vi "lib1.vi"() -> ()   [LabVIEW 2013]
panel:
  out "year of study":i32
  out "Month":i32
  out "number":i32
  out "year":i32
  out "date string":string
  out "id number":i32
  out "offset string rollnumber":string
  out "Roll Number string":string
  out "Image Out":T1(plugin-control)
  in  "stop":bool
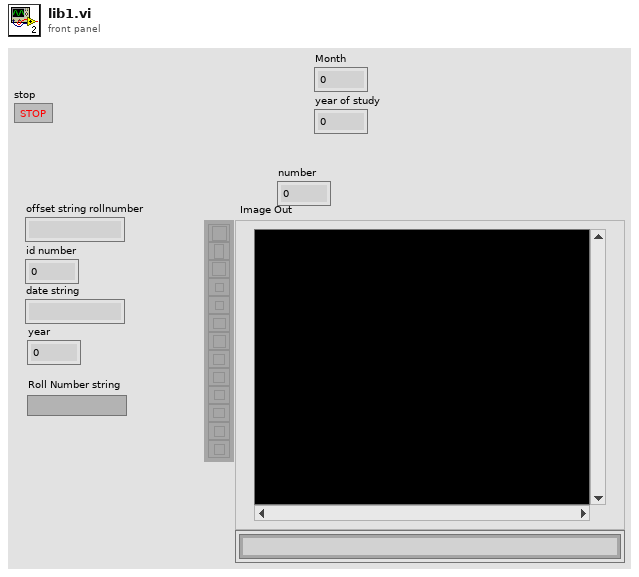
[diagram p1: front panel]
types:
  T1 = typedef "IMAQ Image.ctl" = refnum<image>
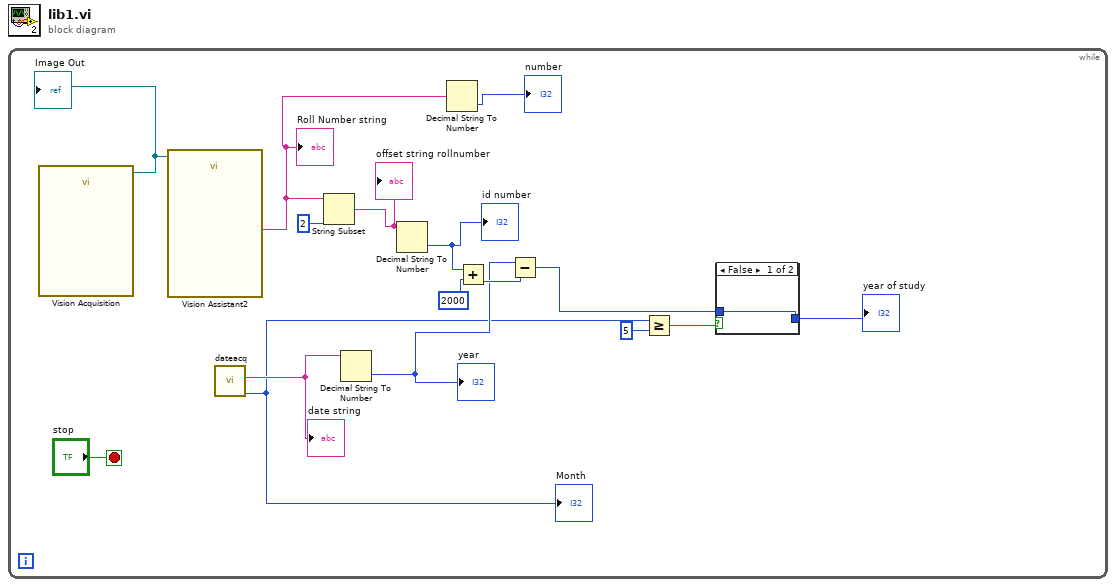
[diagram p0: block diagram]
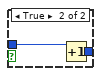
[diagram p2: hidden frame]
diagram:
  n1 = while {
    stop <- "stop" stop-if-true
    n2 = call "Vision Acquisition"() -> ("Image Out"=w16:T1)  [unwired: 24 in, 3 out]
    "Image Out" <- w16
    n3 = call "Vision Assistant2"("Image In"=w16) -> ("String (OCR/OCV 1)"=w6:string)  [unwired: 24 in, 2 out]
    "Roll Number string" <- w6
    n4 = call "dateacq.vi"() -> ("Month"=w5:i32, "substring before match"=w8:string)  [unwired: 8 in, 2 out]
    "date string" <- w8
    "Month" <- w5
    n5 = String Subset(string=w6, length (rest)=2 ("length (rest)")) -> (substring=w13:string)  [unwired: 1 in]
    "offset string rollnumber" <- w13
    n6 = Decimal String To Number(string=w8) -> (number=w9:i32)  [unwired: 2 in, 1 out]
    "year" <- w9
    n7 = Decimal String To Number(string=w13) -> (number=w12:i32)  [unwired: 2 in, 1 out]
    "id number" <- w12
    n8 = Decimal String To Number(string=w6) -> (number=→"number":i32)  [unwired: 2 in, 1 out]
    n9 = Add(x=w12, y=2000) -> (x+y=w10:i32)
    n10 = Subtract(x=w9, y=w10) -> (x-y=w2:i32)
    n11 = Greater Or Equal?(x=w5, y=5) -> (x >= y?=w3:bool)
    n12 = case shown="False" w3 {
      tunnel: w2 -> [w17 w19]
      tunnel: [w17 w18] -> w1
      frame False {
      }
      frame True {
        n13 = Increment(x=w19) -> (x+1=w18:i32)
      }
    }
    "year of study" <- w1
  }
